vi "fgt set purge.vi"(8 "error in (no error)":errorcluster, 10 "purge":bool, 11 "controllerIndex":u16) -> (0 "error out":errorcluster)   [LabVIEW 2020, in "fgt_SDK.lvlib"]
doc: "Activate/deactivate purge function.\nThis feature is only available on MFCS devices equipped with special valve."
uses:
  fgt_SDK.lvlib
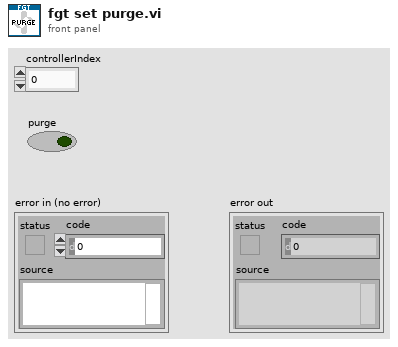
[diagram p1: front panel]
types:
  T1 = typedef "fgt_SDK.lvlib/fgt_STATUS_INFO.ctl" = cluster{"InstrType":T2, "instrSN":u16, "errorCode":u8, "infoCode":u8, "detail":string}
  T2 = typedef "fgt_SDK.lvlib/fgt_INSTRUMENT_TYPE.ctl" = enum32{"None", "MFCS", "MFCS_EZ", "FRP", "LineUP", "IPS"}
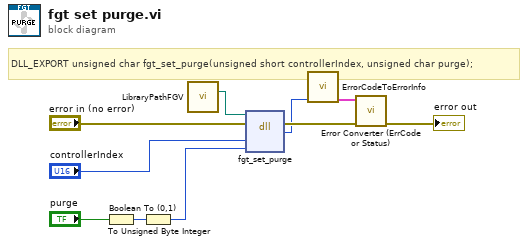
[diagram p0: block diagram]
diagram:
  # "DLL_EXPORT unsigned char fgt_set_purge(unsigned short controllerIndex, unsigned char purge);"
  n1 = Boolean To (0,1)(Boolean="purge") -> (0, 1=w6:i16)
  n2 = To Unsigned Byte Integer(number=w6) -> (unsigned 8bit integer=w4:u8)
  n3 = call "LibraryPathFGV.vi"() -> ("Path Out"=w1:path)  [unwired: 14 in, 1 out]
  n4 = dll-call lib="C:/Workspace/fgt-SDK/LabVIEW/dlls/fgt_SDK_*.*" fn="fgt_set_purge"(path in=w1, error in="error in (no error)", "controllerIndex"="controllerIndex", "purge"=w4) -> (error out=w8:errorcluster, "return type"=w3:u8)  [unwired: 3 in, 1 out]
  n5 = call "ErrorCodeToErrorInfo.vi"("return type"=w3) -> ("StatusInfo"=w2:T1)  [unwired: 10 in]
  n6 = call "Error Converter (ErrCode or Status).vi"("error in (no error)"=w8, "StatusInfo"=w2) -> ("error out"=→"error out":errorcluster)  [unwired: 9 in]
